vi "Controles de relés de prueba actualizados.vi"(7 "Fases 3 y 4":bool, 8 "error in (no error)":errorcluster, 9 "Fases 1 y 2":bool, 10 "Cojinete":bool) -> (0 "error out":errorcluster)   [LabVIEW 2020, in "Pruebas.lvlib"]
doc: "Controles de relés de prueba actualizados\n_____\nCreated using Delacor QMH Event Scripter 5.0.0.112."
uses:
  Pruebas.lvlib
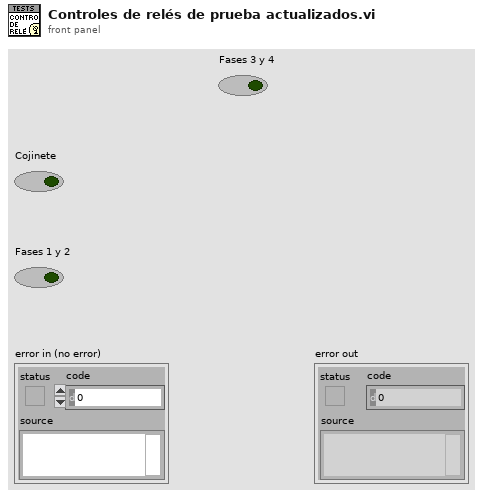
[diagram p1: front panel]
types:
  T1 = typedef "Pruebas.lvlib/Controles de relés de prueba actualizados Argument--cluster.ctl" = cluster{"Cojinete":bool, "Fases 1 y 2":bool, "Fases 3 y 4":bool}
  T2 = typedef "Pruebas.lvlib/Broadcast Events--cluster.ctl" = cluster{"Module Did Init":refnum<user-event>, "Status Updated":refnum<user-event>, "Error Reported":refnum<user-event>, "Module Did Stop":refnum<user-event>, "Update Module Execution Status":refnum<user-event>, "Controles de relés de prueba actualizados":refnum<user-event>, "Valor de Medicion de Prueba Enviado":refnum<user-event>, "Valor de Modulacion Debugging Enviado":refnum<user-event>}
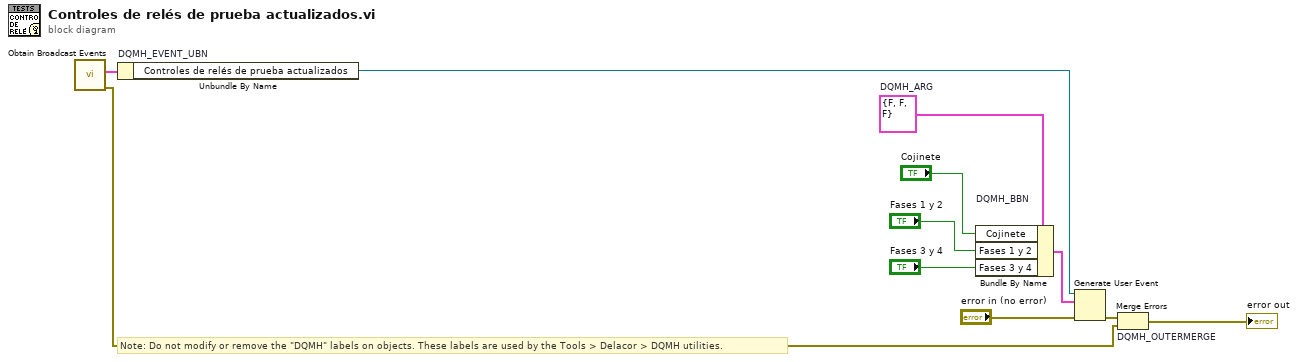
[diagram p0: block diagram]
diagram:
  w6 = T1 {"Cojinete"=FALSE, "Fases 1 y 2"=FALSE, "Fases 3 y 4"=FALSE}  # DQMH_ARG
  # "Note: Do not modify or remove the \"DQMH\" labels on objects. These labels are used by the Tools > Delacor > DQMH utilities."
  n1 = call "Obtain Broadcast Events.vi"() -> ("error out"=w2:errorcluster, "Pruebas Broadcast Events"=w1:T2)  [unwired: 10 in]
  n2 = Unbundle By Name "DQMH_EVENT_UBN"(w1) -> ("Controles de relés de prueba actualizados"=w8:refnum<user-event>)
  n3 = Bundle By Name "DQMH_BBN"(cluster=w6, "Cojinete"="Cojinete", "Fases 1 y 2"="Fases 1 y 2", "Fases 3 y 4"="Fases 3 y 4") -> (w9:T1)
  n4 = Generate User Event(user event=w8, event data cluster=w9, error in="error in (no error)") -> (error out=w7:errorcluster)  [unwired: 1 in, 1 out]
  n5 = Merge Errors "DQMH_OUTERMERGE"(w7, w2) -> (→"error out":errorcluster)
